vi "residues of one root.vi"(8 "multiplicity of root":i32, 9 "root":cdb format="%#_4g", 10 "Denominator":cdb[](array[numeric]) format="%#.2g", 11 "Rest":cdb[](array[numeric]) format="%#.2g") -> (3 "Residues of root":cdb[](array[numeric]) format="%#_4g")   [LabVIEW 2010, in "NI_AALPro.lvlib"]
uses:
  NI_AALPro.lvlib
  Divide Polynomials (CDB).vi
  NI_Gmath.lvlib
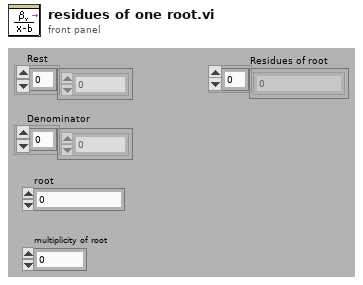
[diagram p1: front panel]
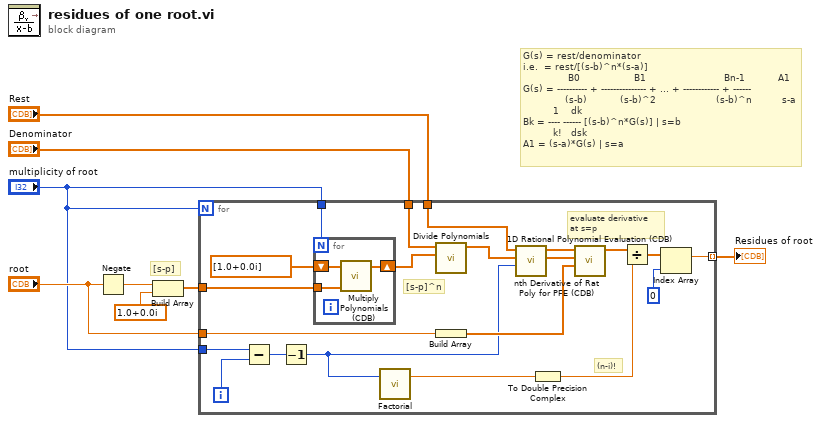
[diagram p0: block diagram]
diagram:
  # "G(s) = rest/denominator   \ni.e.  = rest/[(s-b)^n*(s-a)]\n               B0                  B1                          Bn-1           A1\nG(s) = ---------- + --------------- + ... + ------------ + ------\n              (s-b)           (s-b)^2                    (s-b)^n          s-a\n          1    dk\nBk = ---- ------ [(s-b)^n*G(s)] | s=b \n          k!   dsk\nA1 = (s-a)*G(s) | s=a"
  # "[s-p]"
  n1 = Negate(x="root") -> (-x=w5:cdb)
  n2 = Build Array(w5, cdb 1.0+0.0i) -> (w4:cdb[])
  n3 = for {
    N: "multiplicity of root" -> [_]
    tunnel: "multiplicity of root" -> [w27]
    tunnel: w4 -> [w28]
    tunnel: "Denominator" -> [w11]
    tunnel: "root" -> [w20]
    tunnel: [w18] -> w1 mode=indexing
    tunnel: "multiplicity of root" -> [w25]
    tunnel: "Rest" -> [w12]
    i -> [w24]
    # "(n-i)!"
    # "[s-p]^n"
    # "evaluate derivative\nat s=p"
    n4 = Subtract(x=w27, y=w24) -> (x-y=w23:i32)
    n5 = Decrement(x=w23) -> (x-1=w14:i32)
    n6 = for {
      N: w25 -> [_]
      shift-right: [w31] -> w10
      shift-left: cdb[] [1.0+0.0i] ("p*q") -> [w32]
      tunnel: w28 -> [w30]
      n7 = call "Multiply Polynomials (CDB).vi"("Q(x)"=w30, "P(x)"=w32) -> ("P(x)*Q(x)"=w31:cdb[])  [unwired: 8 in, 1 out]
    }
    n8 = call "Factorial.vi"("n"=w14) -> ("n!"=w13:dbl)  [unwired: 2 in]
    n9 = call-poly "Divide Polynomials.vi"("Q(x)"=w10, "P(x)"=w11) -> ("P(x)/Q(x)"=w9:cdb[])  [unwired: 7 in, 2 out]
    n10 = Build Array(w20) -> (w16:cdb[])
    n11 = call "nth Derivative of Rat Poly for PFE (CDB).vi"("order"=w14, "Q(x)"=w9, "P(x)"=w12) -> ("Denominator d[P(x)/Q(x)]/dx"=w21:cdb[], "Numerator d[P(x)/Q(x)]/dx"=w22:cdb[])  [unwired: 6 in, 1 out]
    n12 = To Double Precision Complex(1:w13) -> (0:w26:cdb)
    n13 = call "1D Rational Polynomial Evaluation (CDB).vi"("A"=w16, "Q(x)"=w21, "P(x)"=w22) -> ("P(A)/Q(A)"=w15:cdb[])  [unwired: 7 in, 1 out]
    n14 = Divide(x=w15, y=w26) -> (x/y=w19:cdb[])
    n15 = Index Array(array=w19, index=0) -> (element=w18:cdb)
  }
  "Residues of root" <- w1
